vi "AI Clear.vi"(11 "clear":bool) -> ()   [LabVIEW 2023]
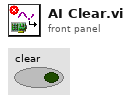
[diagram p1: front panel]
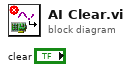
[diagram p0: block diagram]
diagram:
